vi "Read library name.vi"(8 "error in":errorcluster, 11 "editorscriptingobject in":refnum<class "editorscriptingobject.lvclass">) -> (0 "error out":errorcluster, 2 "library name":string, 3 "editorscriptingobject out":refnum<class "editorscriptingobject.lvclass">)   [LabVIEW 2014, in "editorscriptingobject.lvclass"]
uses:
  editorscriptingobject.lvclass
  editorscriptingobject.lvclass/editorscriptingobject.ctl
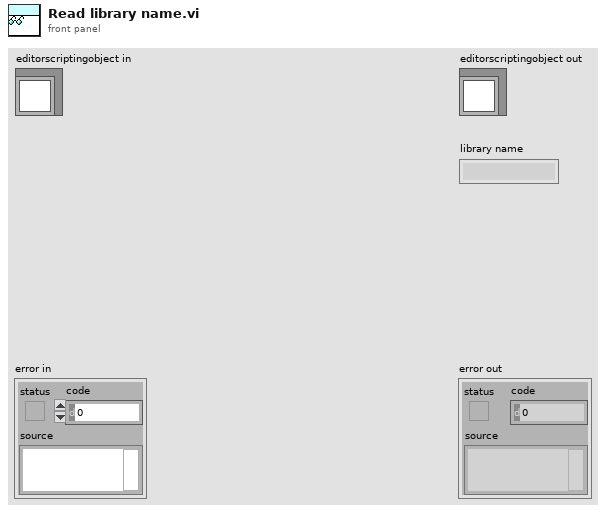
[diagram p1: front panel]
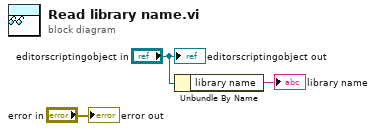
[diagram p0: block diagram]
diagram:
  n1 = Unbundle By Name("editorscriptingobject in") -> ("library name"=→"library name":string)
  "error out" <- "error in"
  "editorscriptingobject out" <- "editorscriptingobject in"
